vi "Inst.RP100.setLevel.vi"(8 "error in (no error)":errorcluster, 10 "Variant":variant, 11 "Inst.RP100 out":refnum<class "Inst.RP100.lvclass">) -> (0 "error out":errorcluster, 3 "Inst.RP100 out":refnum<class "Inst.RP100.lvclass">)   [LabVIEW 2019, in "Inst.RP100.lvlib" / "Inst.RP100.lvclass"]
uses:
  Inst.RP100.lvclass
  Typedefs/State--Enum.ctl
  Typedefs/setLevel--Cluster.ctl
  Typedefs/Channel--Num.ctl
  Inst.RP100.lvclass/Inst.RP100.ctl
  88b0aeda-06b8-4313-b698-33c6c5bebe4b.vi
  88b0aeda-06b8-4313-b698-33c6c5bebe4b.vi/abeb0206-6bb2-4eac-b5ae-b7ebdde2f965.vi
  88b0aeda-06b8-4313-b698-33c6c5bebe4b.vi/13f5bb4a-2f13-440e-87c2-ccd45c96372f.vi
  <vilib>/Utility/Data Type/Get Type Information.vi
  <vilib>/JDP Science/JSONtext/JSON text to Variant.vi
  <vilib>/JDP Science/JSONtext/LVClass Serializer/JSONtext LVClass Serializer.lvclass
  RP100/RP100.lvlib
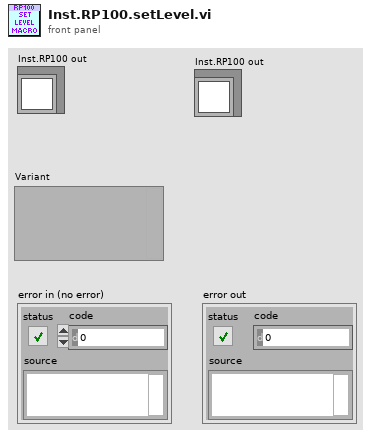
[diagram p1: front panel]
types:
  T1 = typedef "Inst.RP100.lvlib/Inst.RP100.lvclass/setLevel--Cluster.ctl" = cluster{"channel":T2, "level":dbl, "slew":dbl}
  T2 = typedef "Inst.RP100.lvlib/Inst.RP100.lvclass/Channel--Num.ctl" = i32
  T3 = typedef "Inst.RP100.lvlib/Inst.RP100.lvclass/State--Enum.ctl" = enum16{"Shorted", "Enabled"}
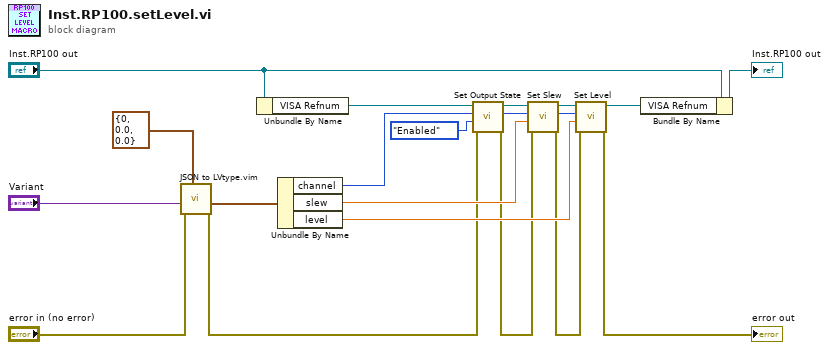
[diagram p0: block diagram]
diagram:
  n1 = call "JSON to LVtype.vim"("type"=T1 {"channel"=0, "level"=0.0, "slew"=0.0} ("Data in"), "error in (no error)"="error in (no error)", "JSON Data in"="Variant") -> ("error out"=w1:errorcluster, "Data out"=w3:T1)  [unwired: 7 in]
  n2 = Unbundle By Name("Inst.RP100 out") -> ("VISA Refnum"=w9:refnum<visa-resource-name>)
  n3 = Unbundle By Name(w3) -> ("channel"=w19:T2, "slew"=w18:dbl, "level"=w20:dbl)
  n4 = call "Set Output State.vi"("error in (no error)"=w1, "Output State"=State--Enum."Enabled", "Output Channel"=w19, "VISA resource name"=w9) -> ("error out"=w11:errorcluster, "Output Channel"=w15:T2, "VISA Refnum out"=w14:refnum<visa-resource-name>)  [unwired: 5 in]
  n5 = call "Set Slew.vi"("error in (no error)"=w11, "Slew (V/s)"=w18, "Output Channel"=w15, "VISA resource name"=w14) -> ("error out"=w12:errorcluster, "Output Channel"=w16:T2, "VISA Refnum out"=w17:refnum<visa-resource-name>)  [unwired: 5 in]
  n6 = call "Set Level.vi"("error in (no error)"=w12, "Level (V)"=w20, "Output Channel"=w16, "VISA resource name"=w17) -> ("error out"=→"error out":errorcluster, "VISA Refnum out"=w8:refnum<visa-resource-name>)  [unwired: 5 in, 1 out]
  n7 = Bundle By Name(cluster="Inst.RP100 out", "VISA Refnum"=w8) -> (→"Inst.RP100 out":refnum<class "Inst.RP100.lvclass">)
